vi "ImportDeviceNames.vi"(1 "PXI card names":string[](array[string])=["DIO:", "6509", "Counter:", "6733_1", "Slow AO:", "6723", "Fast AO:", "6733_1", "6733_2", "6733_3"], 2 "Cleared OK?":errorcluster, 3 "Input Cluster in":T1={"inbits"=8, "outbits"=38, "Counter"="6733_1", "Digital"="6509", "Fast AO"=["6733_1", "6733_2", "6733_3"], "Task Names"=["Inbits", "Outbits", "Counter", "Fast AO_1", "Fast AO_2"]}) -> (0 "Input Cluster out":T1={"inbits"=8, "outbits"=38, "Counter"="6733_1", "Digital"="6509", "Fast AO"=["6733_1", "6733_2", "6733_3"], "Task Names"=["Inbits", "Outbits", "Counter", "FastAO_1", "FastAO_2", "FastAO_3"]})   [LabVIEW 2018]
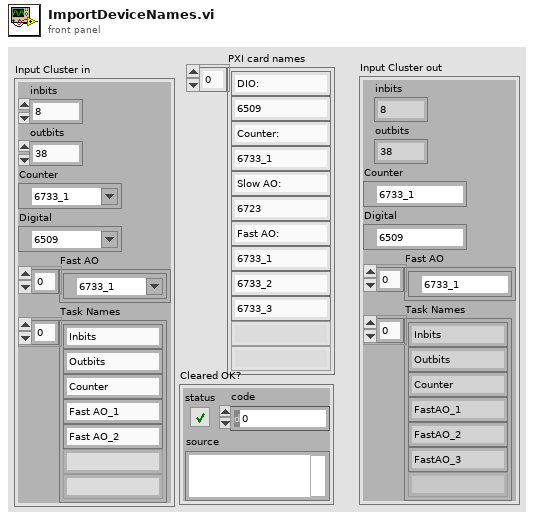
[diagram p1: front panel]
types:
  T1 = cluster{"inbits":i32, "outbits":i32, "Counter":tag, "Digital":tag, "Fast AO":tag[], "Task Names":string[]}
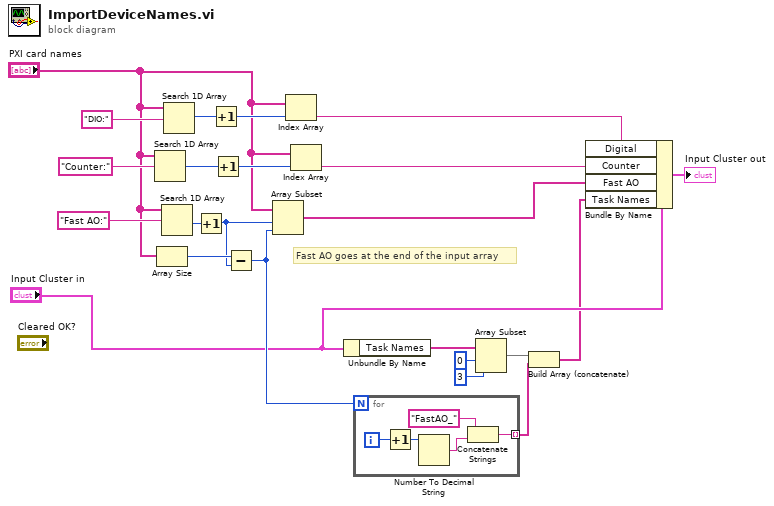
[diagram p0: block diagram]
diagram:
  # "Fast AO goes at the end of the input array"
  n1 = Search 1D Array(1D array="PXI card names", element="Counter:") -> (index of element=w14:i32)  [unwired: 1 in]
  n2 = Array Size(array="PXI card names") -> (size(s)=w12:i32)
  n3 = Search 1D Array(1D array="PXI card names", element="Fast AO:") -> (index of element=w19:i32)  [unwired: 1 in]
  n4 = Search 1D Array(1D array="PXI card names", element="DIO:") -> (index of element=w18:i32)  [unwired: 1 in]
  n5 = Increment(x=w19) -> (x+1=w11:i32)
  n6 = Increment(x=w18) -> (x+1=w16:i32)
  n7 = Increment(x=w14) -> (x+1=w15:i32)
  n8 = Subtract(x=w12, y=w11) -> (x-y=w8:i32)
  n9 = Array Subset(array="PXI card names", index=w11, length=w8) -> (w9:string[])
  n10 = Index Array(array="PXI card names", index=w16) -> (element=w17:string)
  n11 = Index Array(array="PXI card names", index=w15) -> (element=w10:string)
  n12 = Unbundle By Name("Input Cluster in") -> ("Task Names"=w7:string[])
  n13 = for {
    N: w8 -> [_]
    tunnel: [w24] -> w3 mode=indexing
    i -> [w28]
    n14 = Increment(x=w28) -> (x+1=w27:i32)
    n15 = Number To Decimal String(number=w27) -> (decimal integer string=w26:string)  [unwired: 1 in]
    n16 = Concatenate Strings("FastAO_" ("string"), w26) -> (w24:string)
  }
  n17 = Array Subset(array=w7, index=0, length=3) -> (w4:string[])
  n18 = Build Array (concatenate)(w4, w3) -> (w1:string[])
  n19 = Bundle By Name(cluster="Input Cluster in", "Digital"=w17, "Counter"=w10, "Fast AO"=w9, "Task Names"=w1) -> (→"Input Cluster out":T1)
